vi "SaveConfig.vi"(8 "error in (no error)":errorcluster, 11 "GRMActor in":refnum<class "QPDController.lvclass">) -> (0 "error out":errorcluster, 3 "GRMActor out":refnum<class "QPDController.lvclass">)   [LabVIEW 2020, in "QPDController.lvlib" / "QPDController.lvclass"]
uses:
  QPDController.lvclass
  QPDController.lvclass/QPDController.ctl
  Model/Hardware Abstraction Layer/Component/GenericActor/GenericActor/GenericController.lvclass
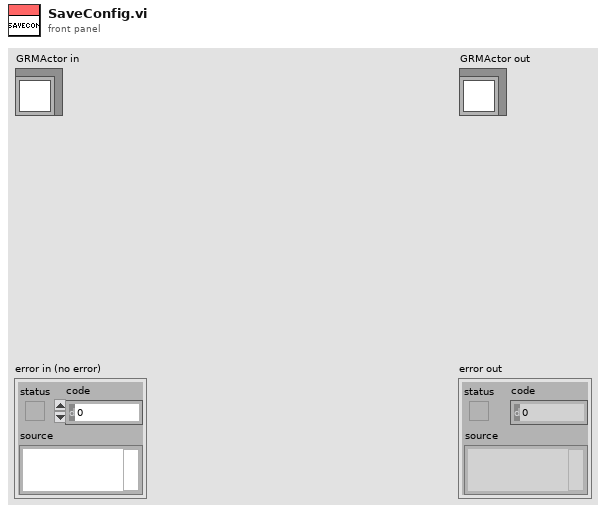
[diagram p1: front panel]
types:
  T1 = typedef "NI_LVConfig.lvlib/Config Data RefNum.ctl" = refnum<k1>
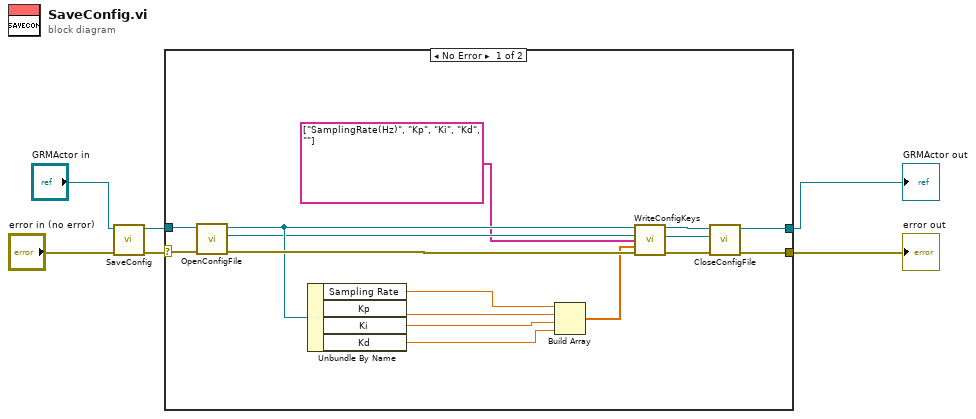
[diagram p0: block diagram]
diagram:
  n1 = call-parent "SaveConfig.vi"("error in (no error)"="error in (no error)", "GRMActor in"="GRMActor in") -> ("error out"=w3:errorcluster, "GRMActor out"=w4:refnum<class "QPDController.lvclass">)  [unwired: 8 in]
  n2 = case shown="No Error" w3 {
    selector: w3 -> [w22 w23]
    tunnel: [w19 w23] -> w1
    tunnel: [w17 w24] -> w2
    tunnel: w4 -> [w16 w24]
    frame No Error {
      n3 = call-dynamic "OpenConfigFile.vi"("error in (no error)"=w22, "GRMActor in"=w16) -> ("error out"=w20:errorcluster, "refnum"=w14:T1, "GRMActor out"=w15:refnum<class "QPDController.lvclass">)  [unwired: 7 in]
      n4 = Unbundle By Name(w15) -> ("Sampling Rate"=w12:dbl, "Kp"=w11:dbl, "Ki"=w10:dbl, "Kd"=w9:dbl)
      n5 = Build Array(w12, w11, w10, w9) -> (w8:dbl[])
      n6 = call-dynamic "WriteConfigKeys.vi"("GRMActor in"=w15, "Config Refnum"=w14, "Keys"=string[] ["SamplingRate(Hz)", "Kp", "Ki", "Kd", ""] ("Values"), "DoubleValue"=w8, "error in (no error)"=w20) -> ("GRMActor out"=w18:refnum<class "QPDController.lvclass">, "Config Refnum dup"=w13:T1, "error out"=w21:errorcluster)  [unwired: 8 in]
      n7 = call-dynamic "CloseConfigFile.vi"("error in (no error)"=w21, "refnum"=w13, "GRMActor in"=w18) -> ("error out"=w19:errorcluster, "GRMActor out"=w17:refnum<class "QPDController.lvclass">)  [unwired: 7 in]
    }
    frame Error {
    }
  }
  "error out" <- w1
  "GRMActor out" <- w2
